vi "File_Write_v2.vi"(0 "Thermocouple Data":dynamicdata(waveform), 1 "Pressure Data":T2, 3 "Flow Rate Data":cluster{dbl, dbl, dbl, dbl, dbl}, 4 "Raman Data Array":cluster{i32[], i32[]}[](array[cluster]), 5 "Loop Iteration Boolean":bool, 8 "File Path Cluster":T3, 9 "Data Cluster":T1={"Current DoE"=[], "SSI 1 Flow Rate"=0.0, "SSI 2 Flow Rate"=0.0, "FLOM 1 Flow Rate"=0.0, "FLOM 2 Flow Rate"=0.0, "Pumps Running?"=FALSE, "Boolean 2"=FALSE, "Boolean 3"=FALSE, "Boolean 4"=FALSE, "At Equilibrium?"=FALSE, "Script Running?"=FALSE, "Current Script Iteration"=0.0, "Total Script Iterations"=0.0, "FLOM Pumps VISA"="COM2", "SSI 1 Pump VISA"="COM76", "SSI 2 Pump VISA"="COM74", "Huber Unistat VISA"="COM1", "SSI 3 Pump VISA"="COM76", "SSI 4 Pump VISA"="COM76", "SSI 4 Flow Rate"=0.0, "SSI 3 Flow Rate"=0.0, "Flow Meter 1"="COM76", "Flow Meter 2"="COM76", "Flow Meter 3"="COM76", "Flow Meter 4"="COM76", "Flow Meter 1 Rate "=0.0, "Flow Meter 2 Rate"=0.0, "Flow Meter 3 Rate"=0.0, "Flow Meter 4 Rate"=0.0, "SSI 1 Flow Setpoint"=0.0, "SSI 2 Flow Setpoint"=0.0, "SSI 3 Flow Setpoint"=0.0, "SSI 4 Flow Setpoint"=0.0, "Temperature Setpoint"=0.0} {"Current DoE" format="%0.3f"}, 12 "Numeric":i32, 13 "Array":i32[](array[numeric])) -> (14 "Data_noRaman path":path, 15 "Data_Reactant 1 path":path caption="selected path", 16 "Data_Reactant 1 path":path, 17 "Data_Reactant 2 path":path caption="selected path", 20 "Data_Reactant 2 path":path, 21 "Data_Reactant 3 path":path, 23 "Data_Product path":path, 24 "Data_noRaman path":path caption="selected path", 25 "Data_Product path":path caption="selected path", 27 "Data_Reactant 3 path":path caption="selected path")   [LabVIEW 2015]
uses:
  --Controls and TypeDefs--/DoE_Control_Cluster.ctl
  <vilib>/Utility/file.llb/Write To Spreadsheet File (string).vi
panel:
  out "appended array":dbl[](array[numeric])
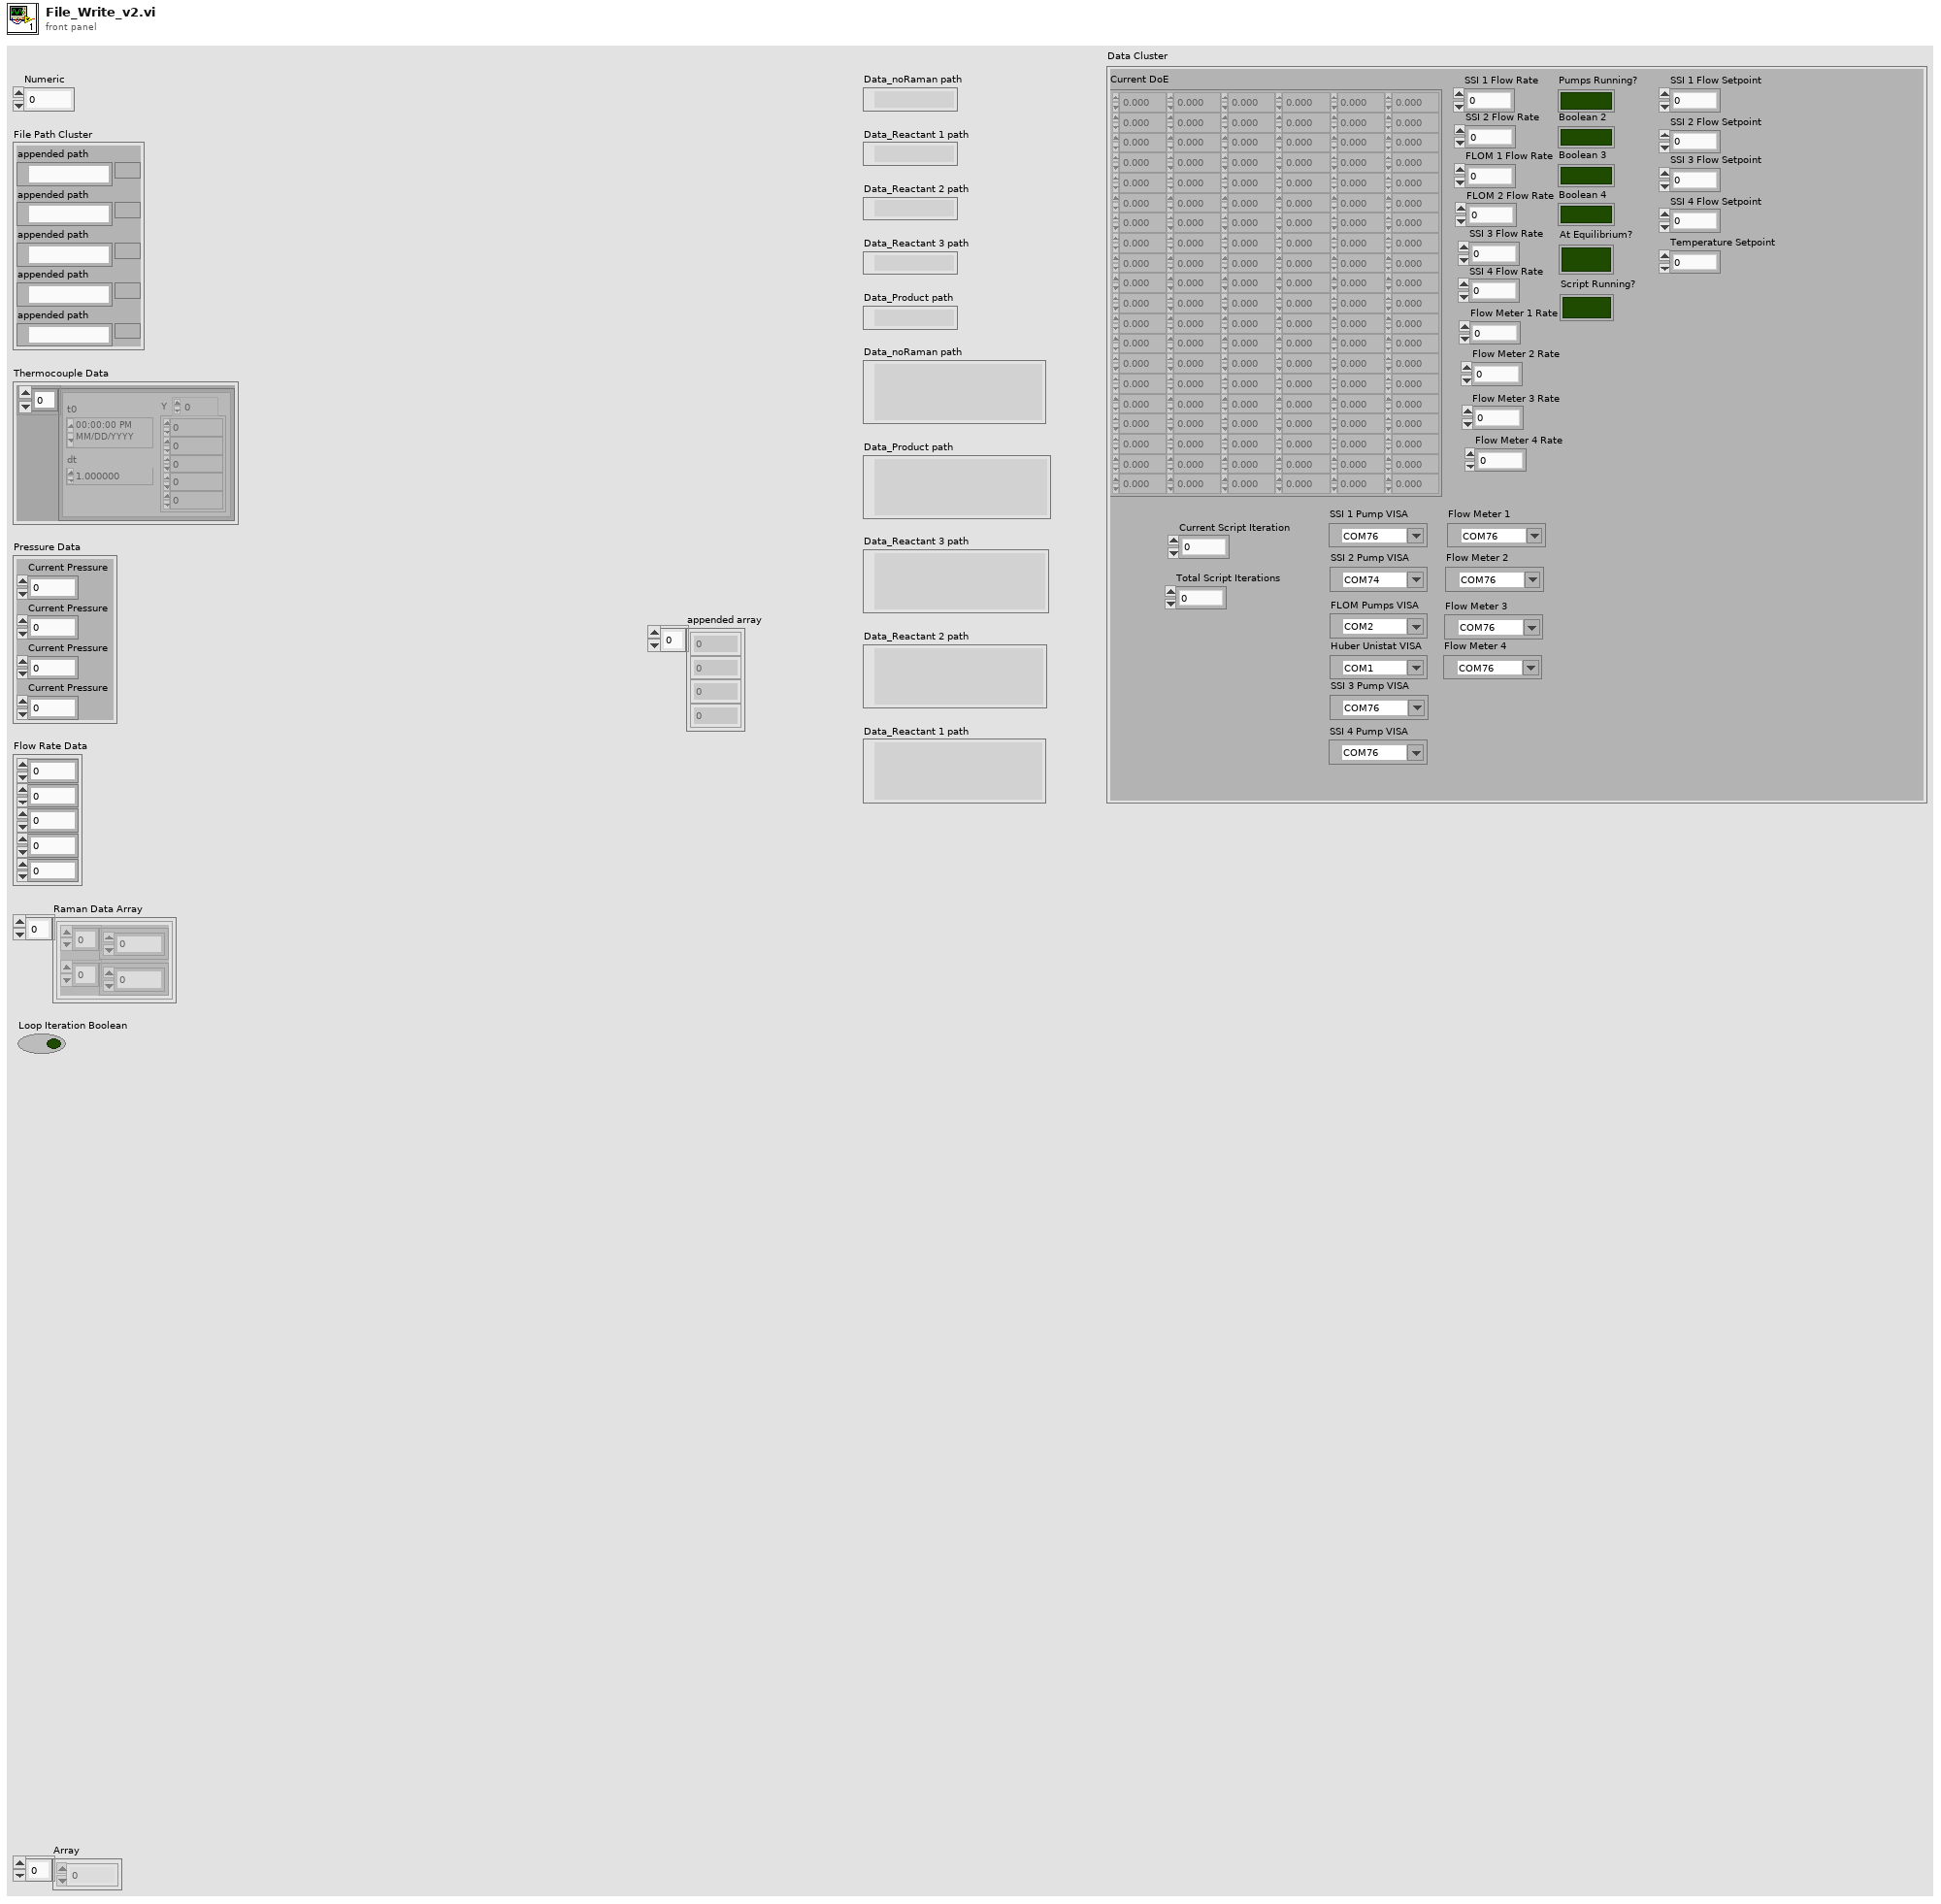
[diagram p1: front panel]
types:
  T1 = typedef "DoE_Control_Cluster.ctl" = cluster{"Current DoE":dbl[][], "SSI 1 Flow Rate":dbl, "SSI 2 Flow Rate":dbl, "FLOM 1 Flow Rate":dbl, "FLOM 2 Flow Rate":dbl, "Pumps Running?":bool, "Boolean 2":bool, "Boolean 3":bool, "Boolean 4":bool, "At Equilibrium?":bool, "Script Running?":bool, "Current Script Iteration":dbl, "Total Script Iterations":dbl, "FLOM Pumps VISA":refnum<visa-resource-name>, "SSI 1 Pump VISA":refnum<visa-resource-name>, "SSI 2 Pump VISA":refnum<visa-resource-name>, "Huber Unistat VISA":refnum<visa-resource-name>, "SSI 3 Pump VISA":refnum<visa-resource-name>, "SSI 4 Pump VISA":refnum<visa-resource-name>, "SSI 4 Flow Rate":dbl, "SSI 3 Flow Rate":dbl, "Flow Meter 1":refnum<visa-resource-name>, "Flow Meter 2":refnum<visa-resource-name>, "Flow Meter 3":refnum<visa-resource-name>, "Flow Meter 4":refnum<visa-resource-name>, "Flow Meter 1 Rate ":dbl, "Flow Meter 2 Rate":dbl, "Flow Meter 3 Rate":dbl, "Flow Meter 4 Rate":dbl, "SSI 1 Flow Setpoint":dbl, "SSI 2 Flow Setpoint":dbl, "SSI 3 Flow Setpoint":dbl, "SSI 4 Flow Setpoint":dbl, "Temperature Setpoint":dbl}
  T2 = cluster{"Current Pressure":dbl, "Current Pressure":dbl, "Current Pressure":dbl, "Current Pressure":dbl}
  T3 = cluster{"appended path":path, "appended path":path, "appended path":path, "appended path":path, "appended path":path}
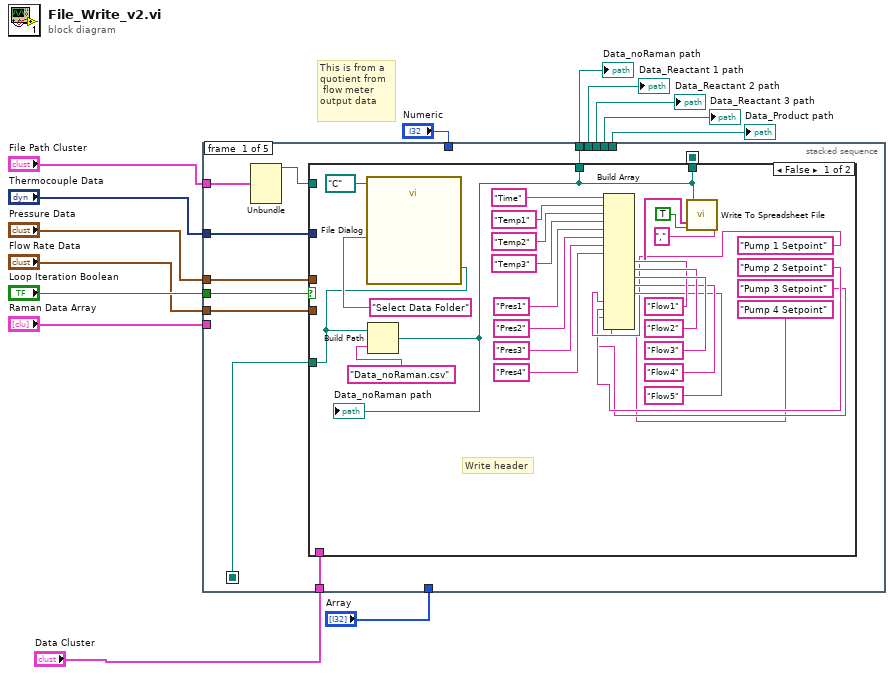
[diagram p0: block diagram]
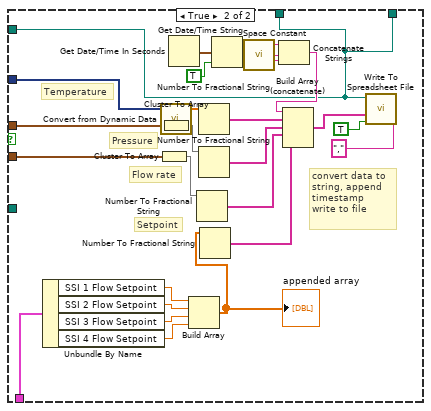
[diagram p2: hidden frame]
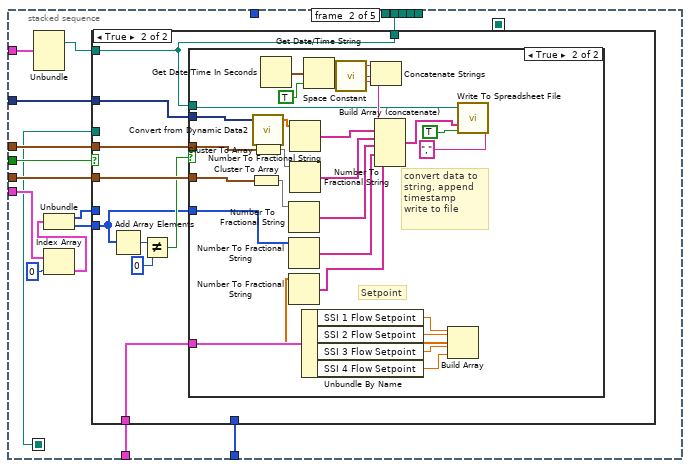
[diagram p3: hidden frame]
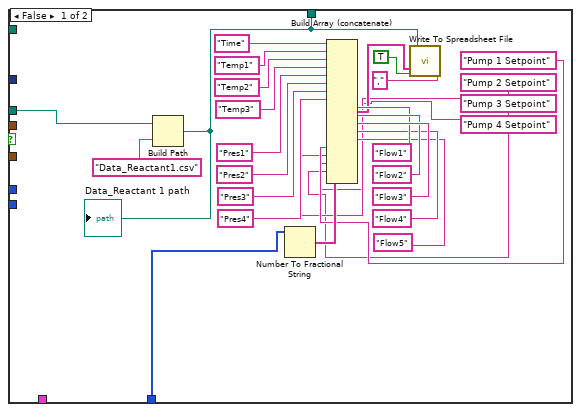
[diagram p4: hidden frame]
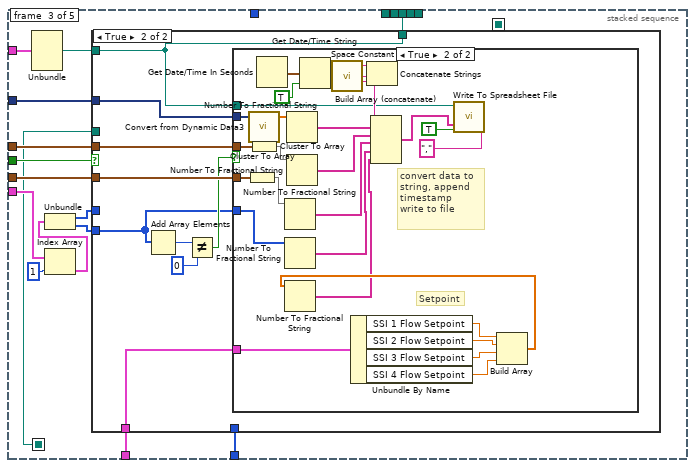
[diagram p6: hidden frame]
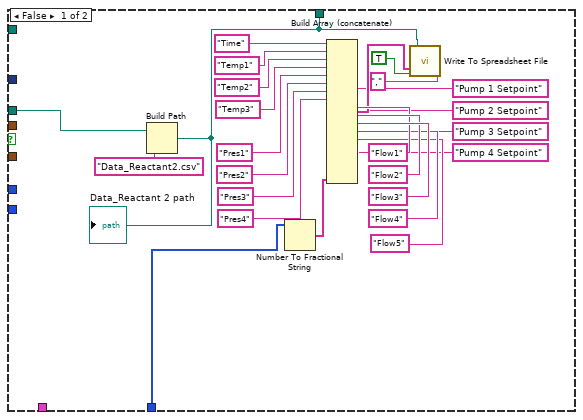
[diagram p7: hidden frame]
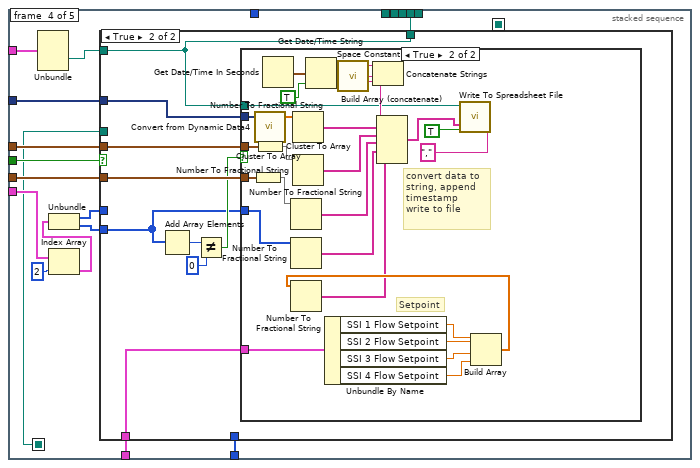
[diagram p9: hidden frame]
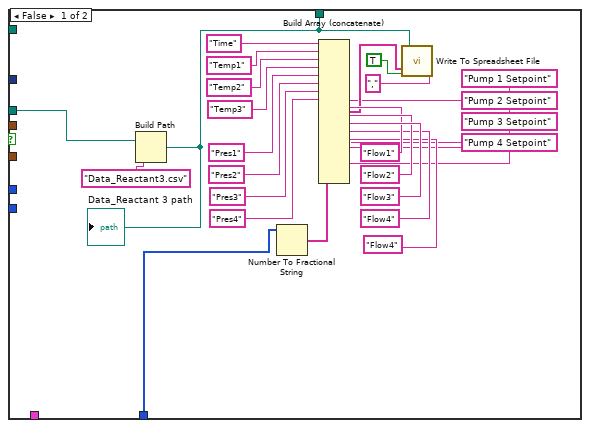
[diagram p10: hidden frame]
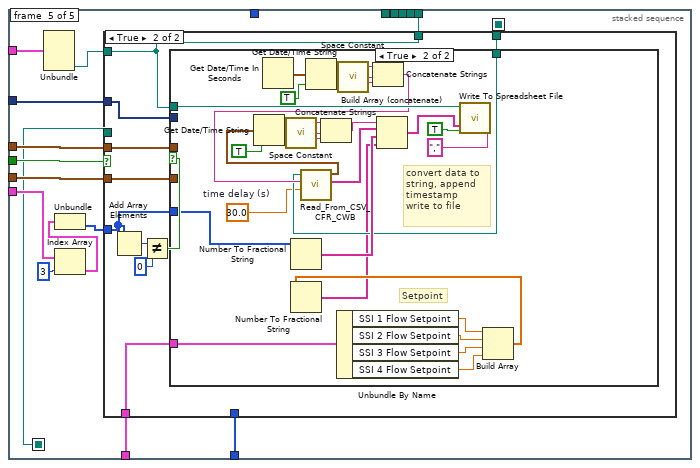
[diagram p12: hidden frame]
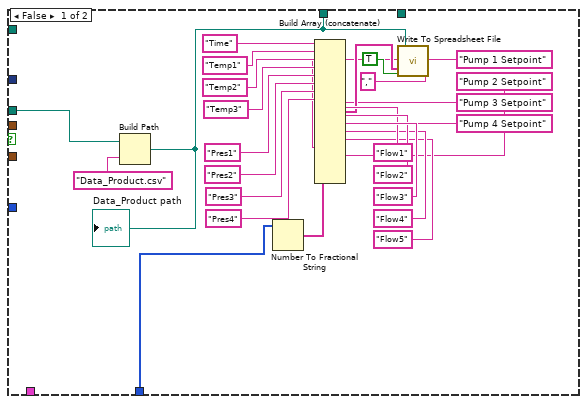
[diagram p13: hidden frame]
diagram:
  # "This is from a \nquotient from\n flow meter\noutput data"
  n1 = stacked-sequence {
    seq-local: [w18 _ _ _ _] -> [_ w78 w155 w232 w310]
    seq-local: [w17 _ _ _ _] -> [_ _ _ _ w308]
    tunnel: "Thermocouple Data" -> [w19 w90 w167 w244 w321]
    tunnel: "Pressure Data" -> [w24 w89 w166 w243 w320]
    tunnel: "Flow Rate Data" -> [w23 w88 w165 w242 w319]
    tunnel: "Loop Iteration Boolean" -> [w22 w87 w164 w241 w318]
    tunnel: [w15 _ _ _ _] -> w12
    tunnel: "File Path Cluster" -> [w21 w80 w157 w234 w312]
    tunnel: "Raman Data Array" -> [_ w84 w161 w238 w316]
    tunnel: [_ w81 _ _ _] -> w11
    tunnel: [_ _ w158 _ _] -> w10
    tunnel: [_ _ _ w235 _] -> w9
    tunnel: [_ _ _ _ w313] -> w8
    tunnel: "Array" -> [_ w77 w154 w231 w309]
    tunnel: "Numeric" -> [_ _ _ _ _]
    tunnel: "Data Cluster" -> [w16 w76 w153 w230 w307]
    frame #0 {
      n2 = Unbundle(w21) -> ("appended path"=w20:path)  [unwired: 4 out]
      n3 = case shown="False" w22 {
        tunnel: w19 -> [_ w63]
        tunnel: w24 -> [_ w62]
        tunnel: w23 -> [_ w59]
        tunnel: w20 -> [_ w57]
        tunnel: [w30 w57] -> w15
        tunnel: [w31 _] -> w18
        tunnel: [w30 w57] -> w17
        tunnel: w16 -> [_ w56]
        frame False {
          # "Write header"
          n4 = call "File Dialog"("start path"=path "C:/", "prompt"="Select Data Folder") -> ("selected path"=w31:path)  [unwired: 10 in, 3 out]
          n5 = Build Path(base path=w31, name or relative path="Data_noRaman.csv" ("default name")) -> (appended path=w30:path)
          "Data_noRaman path" <- w30
          n6 = Build Array("Time" ("delimiter (\\t)"), "Temp1" ("delimiter (\\t)"), "Temp2" ("delimiter (\\t)"), "Temp3" ("delimiter (\\t)"), "Pres1" ("delimiter (\\t)"), "Pres2" ("delimiter (\\t)"), "Pres3" ("delimiter (\\t)"), "Pres4" ("delimiter (\\t)"), "Flow1" ("delimiter (\\t)"), "Flow2" ("delimiter (\\t)"), "Flow3" ("delimiter (\\t)"), "Flow4" ("delimiter (\\t)"), "Flow5" ("delimiter (\\t)"), "Pump 1 Setpoint", "Pump 2 Setpoint", "Pump 3 Setpoint", "Pump 4 Setpoint") -> (w37:string[])
          n7 = call-poly <vilib>:"Write To Spreadsheet File.vi"("delimiter (\\t)"="," ("delimiter (\\t)"), "append to file? (new file:F)"=TRUE ("append to file?"), "1D data"=w37, "file path (dialog if empty)"=w30) -> ()  [unwired: 4 in, 1 out]
        }
        frame True {
          # "Setpoint"
          # "Temperature"
          # "Pressure"
          # "Flow rate"
          # "convert data to \nstring, append\ntimestamp\nwrite to file"
          n8 = Unbundle By Name(w56) -> ("SSI 1 Flow Setpoint"=w55:dbl, "SSI 2 Flow Setpoint"=w54:dbl, "SSI 3 Flow Setpoint"=w53:dbl, "SSI 4 Flow Setpoint"=w52:dbl)
          n9 = Cluster To Array(cluster=w59) -> (array=w60:dbl[])
          n10 = call "Convert from Dynamic Data"("Dynamic Data Type"=w63) -> ("Array"=w72:dbl[])  [unwired: 3 in]
          n11 = Cluster To Array(cluster=w62) -> (array=w73:dbl[])
          n12 = Get Date/Time In Seconds() -> (seconds since 1Jan1904=w66:timestamp)
          n13 = Build Array(w55, w54, w53, w52) -> (w51:dbl[])
          "appended array" <- w51
          n14 = Number To Fractional String(number=w60) -> (F-format string=w58:string[])  [unwired: 3 in]
          n15 = Number To Fractional String(number=w72) -> (F-format string=w74:string[])  [unwired: 3 in]
          n16 = Number To Fractional String(number=w73) -> (F-format string=w61:string[])  [unwired: 3 in]
          n17 = Number To Fractional String(number=w51) -> (F-format string=w50:string[])  [unwired: 3 in]
          n18 = Get Date/Time String(seconds (now)=w66, want seconds? (F)=TRUE) -> (date string=w68:string, time string=w69:string)  [unwired: 1 in]
          n19 = call <vilib>:"Space Constant.vi"() -> ("String"=w70:string)
          n20 = Concatenate Strings(w68, w70, w69) -> (w71:string)
          n21 = Build Array (concatenate)(w71, w74, w61, w58, w50) -> (w75:string[])
          n22 = call-poly <vilib>:"Write To Spreadsheet File.vi"("delimiter (\\t)"="," ("delimiter (\\t)"), "append to file? (new file:F)"=TRUE ("append to file?"), "1D data"=w75, "file path (dialog if empty)"=w57) -> ()  [unwired: 4 in, 1 out]
        }
      }
    }
    frame #1 {
      n23 = Unbundle(w80) -> ("appended path"=w79:path)  [unwired: 4 out]
      n24 = Index Array(array=w84, index=0) -> (element=w83:cluster{i32[], i32[]})
      n25 = Unbundle(w83) -> (w85:i32[], w86:i32[])
      n26 = case shown="True" w87 {
        tunnel: w90 -> [_ w124]
        tunnel: w89 -> [_ w123]
        tunnel: w88 -> [_ w122]
        tunnel: w79 -> [_ w121]
        tunnel: [w115 w121] -> w81
        tunnel: w86 -> [_ w117]
        tunnel: w85 -> [_ _]
        tunnel: w78 -> [w114 _]
        tunnel: w77 -> [w97 _]
        tunnel: w76 -> [_ w116]
        frame False {
          n27 = Build Path(base path=w114, name or relative path="Data_Reactant1.csv" ("default name")) -> (appended path=w115:path)
          "Data_Reactant 1 path" <- w115
          n28 = Number To Fractional String(number=w97) -> (F-format string=w95:string[])  [unwired: 3 in]
          n29 = Build Array (concatenate)("Time" ("delimiter (\\t)"), "Temp1" ("delimiter (\\t)"), "Temp2" ("delimiter (\\t)"), "Temp3" ("delimiter (\\t)"), "Pres1" ("delimiter (\\t)"), "Pres2" ("delimiter (\\t)"), "Pres3" ("delimiter (\\t)"), "Pres4" ("delimiter (\\t)"), "Flow1" ("delimiter (\\t)"), "Flow2" ("delimiter (\\t)"), "Flow3" ("delimiter (\\t)"), "Flow4" ("delimiter (\\t)"), "Flow5" ("delimiter (\\t)"), "Pump 1 Setpoint", "Pump 2 Setpoint", "Pump 3 Setpoint", "Pump 4 Setpoint", w95) -> (w101:string[])
          n30 = call-poly <vilib>:"Write To Spreadsheet File.vi"("delimiter (\\t)"="," ("delimiter (\\t)"), "append to file? (new file:F)"=TRUE ("append to file?"), "1D data"=w101, "file path (dialog if empty)"=w115) -> ()  [unwired: 4 in, 1 out]
        }
        frame True {
          n31 = Add Array Elements(numeric array=w117) -> (sum=w120:i32)
          n32 = Not Equal?(x=w120, y=0) -> (x != y?=w118:bool)
          n33 = case shown="True" w118 {
            tunnel: w124 -> [_ w140]
            tunnel: w123 -> [_ w139]
            tunnel: w122 -> [_ w136]
            tunnel: w121 -> [_ w134]
            tunnel: w117 -> [_ w133]
            tunnel: w116 -> [_ w128]
            frame False {
            }
            frame True {
              # "Setpoint"
              # "convert data to \nstring, append\ntimestamp\nwrite to file"
              n34 = Cluster To Array(cluster=w136) -> (array=w137:dbl[])
              n35 = call "Convert from Dynamic Data2"("Dynamic Data Type"=w140) -> ("Array"=w149:dbl[])  [unwired: 3 in]
              n36 = Cluster To Array(cluster=w139) -> (array=w150:dbl[])
              n37 = Get Date/Time In Seconds() -> (seconds since 1Jan1904=w143:timestamp)
              n38 = Number To Fractional String(number=w137) -> (F-format string=w135:string[])  [unwired: 3 in]
              n39 = Number To Fractional String(number=w133) -> (F-format string=w132:string[])  [unwired: 3 in]
              n40 = Number To Fractional String(number=w149) -> (F-format string=w151:string[])  [unwired: 3 in]
              n41 = Number To Fractional String(number=w150) -> (F-format string=w138:string[])  [unwired: 3 in]
              n42 = Unbundle By Name(w128) -> ("SSI 1 Flow Setpoint"=w131:dbl, "SSI 2 Flow Setpoint"=w127:dbl, "SSI 3 Flow Setpoint"=w130:dbl, "SSI 4 Flow Setpoint"=w129:dbl)
              n43 = Get Date/Time String(seconds (now)=w143, want seconds? (F)=TRUE) -> (date string=w145:string, time string=w146:string)  [unwired: 1 in]
              n44 = call <vilib>:"Space Constant.vi"() -> ("String"=w147:string)
              n45 = Concatenate Strings(w145, w147, w146) -> (w148:string)
              n46 = Build Array(w131, w127, w130, w129) -> (w126:dbl[])
              n47 = Number To Fractional String(number=w126) -> (F-format string=w125:string[])  [unwired: 3 in]
              n48 = Build Array (concatenate)(w148, w151, w138, w135, w132, w125) -> (w152:string[])
              n49 = call-poly <vilib>:"Write To Spreadsheet File.vi"("delimiter (\\t)"="," ("delimiter (\\t)"), "append to file? (new file:F)"=TRUE ("append to file?"), "1D data"=w152, "file path (dialog if empty)"=w134) -> ()  [unwired: 4 in, 1 out]
            }
          }
        }
      }
    }
    frame #2 {
      n50 = Unbundle(w157) -> ("appended path"=w156:path)  [unwired: 4 out]
      n51 = Index Array(array=w161, index=1) -> (element=w160:cluster{i32[], i32[]})
      n52 = Unbundle(w160) -> (w162:i32[], w163:i32[])
      n53 = case shown="True" w164 {
        tunnel: w167 -> [_ w201]
        tunnel: w166 -> [_ w200]
        tunnel: w165 -> [_ w199]
        tunnel: w156 -> [_ w198]
        tunnel: [w192 w198] -> w158
        tunnel: w163 -> [_ w194]
        tunnel: w162 -> [_ _]
        tunnel: w155 -> [w191 _]
        tunnel: w154 -> [w174 _]
        tunnel: w153 -> [_ w193]
        frame False {
          n54 = Build Path(base path=w191, name or relative path="Data_Reactant2.csv" ("default name")) -> (appended path=w192:path)
          "Data_Reactant 2 path" <- w192
          n55 = Number To Fractional String(number=w174) -> (F-format string=w172:string[])  [unwired: 3 in]
          n56 = Build Array (concatenate)("Time" ("delimiter (\\t)"), "Temp1" ("delimiter (\\t)"), "Temp2" ("delimiter (\\t)"), "Temp3" ("delimiter (\\t)"), "Pres1" ("delimiter (\\t)"), "Pres2" ("delimiter (\\t)"), "Pres3" ("delimiter (\\t)"), "Pres4" ("delimiter (\\t)"), "Flow1" ("delimiter (\\t)"), "Flow2" ("delimiter (\\t)"), "Flow3" ("delimiter (\\t)"), "Flow4" ("delimiter (\\t)"), "Flow5" ("delimiter (\\t)"), "Pump 1 Setpoint", "Pump 2 Setpoint", "Pump 3 Setpoint", "Pump 4 Setpoint", w172) -> (w178:string[])
          n57 = call-poly <vilib>:"Write To Spreadsheet File.vi"("delimiter (\\t)"="," ("delimiter (\\t)"), "append to file? (new file:F)"=TRUE ("append to file?"), "1D data"=w178, "file path (dialog if empty)"=w192) -> ()  [unwired: 4 in, 1 out]
        }
        frame True {
          n58 = Add Array Elements(numeric array=w194) -> (sum=w197:i32)
          n59 = Not Equal?(x=w197, y=0) -> (x != y?=w195:bool)
          n60 = case shown="True" w195 {
            tunnel: w201 -> [_ w217]
            tunnel: w200 -> [_ w216]
            tunnel: w199 -> [_ w213]
            tunnel: w198 -> [_ w211]
            tunnel: w194 -> [_ w210]
            tunnel: w193 -> [_ w205]
            frame False {
            }
            frame True {
              # "Setpoint"
              # "convert data to \nstring, append\ntimestamp\nwrite to file"
              n61 = Cluster To Array(cluster=w213) -> (array=w214:dbl[])
              n62 = call "Convert from Dynamic Data3"("Dynamic Data Type"=w217) -> ("Array"=w226:dbl[])  [unwired: 3 in]
              n63 = Cluster To Array(cluster=w216) -> (array=w227:dbl[])
              n64 = Get Date/Time In Seconds() -> (seconds since 1Jan1904=w220:timestamp)
              n65 = Number To Fractional String(number=w214) -> (F-format string=w212:string[])  [unwired: 3 in]
              n66 = Number To Fractional String(number=w210) -> (F-format string=w209:string[])  [unwired: 3 in]
              n67 = Number To Fractional String(number=w226) -> (F-format string=w228:string[])  [unwired: 3 in]
              n68 = Number To Fractional String(number=w227) -> (F-format string=w215:string[])  [unwired: 3 in]
              n69 = Get Date/Time String(seconds (now)=w220, want seconds? (F)=TRUE) -> (date string=w222:string, time string=w223:string)  [unwired: 1 in]
              n70 = call <vilib>:"Space Constant.vi"() -> ("String"=w224:string)
              n71 = Unbundle By Name(w205) -> ("SSI 1 Flow Setpoint"=w208:dbl, "SSI 2 Flow Setpoint"=w204:dbl, "SSI 3 Flow Setpoint"=w207:dbl, "SSI 4 Flow Setpoint"=w206:dbl)
              n72 = Concatenate Strings(w222, w224, w223) -> (w225:string)
              n73 = Build Array(w208, w204, w207, w206) -> (w203:dbl[])
              n74 = Number To Fractional String(number=w203) -> (F-format string=w202:string[])  [unwired: 3 in]
              n75 = Build Array (concatenate)(w225, w228, w215, w212, w209, w202) -> (w229:string[])
              n76 = call-poly <vilib>:"Write To Spreadsheet File.vi"("delimiter (\\t)"="," ("delimiter (\\t)"), "append to file? (new file:F)"=TRUE ("append to file?"), "1D data"=w229, "file path (dialog if empty)"=w211) -> ()  [unwired: 4 in, 1 out]
            }
          }
        }
      }
    }
    frame #3 {
      n77 = Unbundle(w234) -> ("appended path"=w233:path)  [unwired: 4 out]
      n78 = Index Array(array=w238, index=2) -> (element=w237:cluster{i32[], i32[]})
      n79 = Unbundle(w237) -> (w239:i32[], w240:i32[])
      n80 = case shown="True" w241 {
        tunnel: w244 -> [_ w278]
        tunnel: w243 -> [_ w277]
        tunnel: w242 -> [_ w276]
        tunnel: w233 -> [_ w275]
        tunnel: [w269 w275] -> w235
        tunnel: w240 -> [_ w271]
        tunnel: w239 -> [_ _]
        tunnel: w232 -> [w268 _]
        tunnel: w231 -> [w251 _]
        tunnel: w230 -> [_ w270]
        frame False {
          n81 = Build Path(base path=w268, name or relative path="Data_Reactant3.csv" ("default name")) -> (appended path=w269:path)
          "Data_Reactant 3 path" <- w269
          n82 = Number To Fractional String(number=w251) -> (F-format string=w249:string[])  [unwired: 3 in]
          n83 = Build Array (concatenate)("Time" ("delimiter (\\t)"), "Temp1" ("delimiter (\\t)"), "Temp2" ("delimiter (\\t)"), "Temp3" ("delimiter (\\t)"), "Pres1" ("delimiter (\\t)"), "Pres2" ("delimiter (\\t)"), "Pres3" ("delimiter (\\t)"), "Pres4" ("delimiter (\\t)"), "Flow1" ("delimiter (\\t)"), "Flow2" ("delimiter (\\t)"), "Flow3" ("delimiter (\\t)"), "Flow4" ("delimiter (\\t)"), "Flow4" ("delimiter (\\t)"), "Pump 1 Setpoint", "Pump 2 Setpoint", "Pump 3 Setpoint", "Pump 4 Setpoint", w249) -> (w255:string[])
          n84 = call-poly <vilib>:"Write To Spreadsheet File.vi"("delimiter (\\t)"="," ("delimiter (\\t)"), "append to file? (new file:F)"=TRUE ("append to file?"), "1D data"=w255, "file path (dialog if empty)"=w269) -> ()  [unwired: 4 in, 1 out]
        }
        frame True {
          n85 = Add Array Elements(numeric array=w271) -> (sum=w274:i32)
          n86 = Not Equal?(x=w274, y=0) -> (x != y?=w272:bool)
          n87 = case shown="True" w272 {
            tunnel: w278 -> [_ w294]
            tunnel: w277 -> [_ w293]
            tunnel: w276 -> [_ w290]
            tunnel: w275 -> [_ w288]
            tunnel: w271 -> [_ w287]
            tunnel: w270 -> [_ w282]
            frame False {
            }
            frame True {
              # "Setpoint"
              # "convert data to \nstring, append\ntimestamp\nwrite to file"
              n88 = Cluster To Array(cluster=w290) -> (array=w291:dbl[])
              n89 = call "Convert from Dynamic Data4"("Dynamic Data Type"=w294) -> ("Array"=w303:dbl[])  [unwired: 3 in]
              n90 = Cluster To Array(cluster=w293) -> (array=w304:dbl[])
              n91 = Get Date/Time In Seconds() -> (seconds since 1Jan1904=w297:timestamp)
              n92 = Number To Fractional String(number=w291) -> (F-format string=w289:string[])  [unwired: 3 in]
              n93 = Number To Fractional String(number=w287) -> (F-format string=w286:string[])  [unwired: 3 in]
              n94 = Number To Fractional String(number=w303) -> (F-format string=w305:string[])  [unwired: 3 in]
              n95 = Number To Fractional String(number=w304) -> (F-format string=w292:string[])  [unwired: 3 in]
              n96 = Get Date/Time String(seconds (now)=w297, want seconds? (F)=TRUE) -> (date string=w299:string, time string=w300:string)  [unwired: 1 in]
              n97 = Unbundle By Name(w282) -> ("SSI 1 Flow Setpoint"=w285:dbl, "SSI 2 Flow Setpoint"=w279:dbl, "SSI 3 Flow Setpoint"=w284:dbl, "SSI 4 Flow Setpoint"=w283:dbl)
              n98 = call <vilib>:"Space Constant.vi"() -> ("String"=w301:string)
              n99 = Concatenate Strings(w299, w301, w300) -> (w302:string)
              n100 = Build Array(w285, w279, w284, w283) -> (w281:dbl[])
              n101 = Number To Fractional String(number=w281) -> (F-format string=w280:string[])  [unwired: 3 in]
              n102 = Build Array (concatenate)(w302, w305, w292, w289, w286, w280) -> (w306:string[])
              n103 = call-poly <vilib>:"Write To Spreadsheet File.vi"("delimiter (\\t)"="," ("delimiter (\\t)"), "append to file? (new file:F)"=TRUE ("append to file?"), "1D data"=w306, "file path (dialog if empty)"=w288) -> ()  [unwired: 4 in, 1 out]
            }
          }
        }
      }
    }
    frame #4 {
      n104 = Unbundle(w312) -> ("appended path"=w311:path)  [unwired: 4 out]
      n105 = Index Array(array=w316, index=3) -> (element=w315:cluster{i32[], i32[]})
      n106 = Unbundle(w315) -> (w317:i32[])  [unwired: 1 out]
      n107 = case shown="True" w318 {
        tunnel: w321 -> [_ w356]
        tunnel: w320 -> [_ w355]
        tunnel: w319 -> [_ w354]
        tunnel: w311 -> [_ w348]
        tunnel: [w346 w348] -> w313
        tunnel: w317 -> [_ w350]
        tunnel: w310 -> [w345 _]
        tunnel: w309 -> [w328 _]
        tunnel: w308 -> [_ w349]
        tunnel: w307 -> [_ w347]
        frame False {
          n108 = Build Path(base path=w345, name or relative path="Data_Product.csv" ("default name")) -> (appended path=w346:path)
          "Data_Product path" <- w346
          n109 = Number To Fractional String(number=w328) -> (F-format string=w326:string[])  [unwired: 3 in]
          n110 = Build Array (concatenate)("Time" ("delimiter (\\t)"), "Temp1" ("delimiter (\\t)"), "Temp2" ("delimiter (\\t)"), "Temp3" ("delimiter (\\t)"), "Pres1" ("delimiter (\\t)"), "Pres2" ("delimiter (\\t)"), "Pres3" ("delimiter (\\t)"), "Pres4" ("delimiter (\\t)"), "Flow1" ("delimiter (\\t)"), "Flow2" ("delimiter (\\t)"), "Flow3" ("delimiter (\\t)"), "Flow4" ("delimiter (\\t)"), "Flow5" ("delimiter (\\t)"), "Pump 1 Setpoint", "Pump 2 Setpoint", "Pump 3 Setpoint", "Pump 4 Setpoint", w326) -> (w332:string[])
          n111 = call-poly <vilib>:"Write To Spreadsheet File.vi"("delimiter (\\t)"="," ("delimiter (\\t)"), "append to file? (new file:F)"=TRUE ("append to file?"), "1D data"=w332, "file path (dialog if empty)"=w346) -> ()  [unwired: 4 in, 1 out]
        }
        frame True {
          n112 = Add Array Elements(numeric array=w350) -> (sum=w353:i32)
          n113 = Not Equal?(x=w353, y=0) -> (x != y?=w351:bool)
          n114 = case shown="True" w351 {
            tunnel: w356 -> [_ _]
            tunnel: w355 -> [_ _]
            tunnel: w354 -> [_ _]
            tunnel: w348 -> [_ w376]
            tunnel: w350 -> [_ w375]
            tunnel: w349 -> [_ w366]
            tunnel: w347 -> [_ w360]
            frame False {
            }
            frame True {
              w365 = 30.0  # time delay (s)
              # "Setpoint"
              # "convert data to \nstring, append\ntimestamp\nwrite to file"
              n115 = Get Date/Time In Seconds() -> (seconds since 1Jan1904=w379:timestamp)
              n116 = call <vilib>:"Space Constant.vi"() -> ("String"=w373:string)
              n117 = Number To Fractional String(number=w375) -> (F-format string=w367:string[])  [unwired: 3 in]
              n118 = Get Date/Time String(seconds (now)=w379, want seconds? (F)=TRUE) -> (date string=w381:string, time string=w382:string)  [unwired: 1 in]
              n119 = Unbundle By Name(w360) -> ("SSI 1 Flow Setpoint"=w363:dbl, "SSI 2 Flow Setpoint"=w359:dbl, "SSI 3 Flow Setpoint"=w362:dbl, "SSI 4 Flow Setpoint"=w361:dbl)
              n120 = call <vilib>:"Space Constant.vi"() -> ("String"=w383:string)
              n121 = Concatenate Strings(w381, w383, w382) -> (w374:string)
              n122 = call "Read_From_CSV_CFR_CWB.vi"("time delay (s)"=w365, "input string"=w374, "Spreadsheet path (.csv)"=w366) -> ("output data"=w368:string[], "time stamp"=w370:timestamp)  [unwired: 6 in]
              n123 = Get Date/Time String(seconds (now)=w370, want seconds? (F)=TRUE) -> (date string=w364:string, time string=w372:string)  [unwired: 1 in]
              n124 = Concatenate Strings(w364, w373, w372) -> (w369:string)
              n125 = Build Array(w363, w359, w362, w361) -> (w358:dbl[])
              n126 = Number To Fractional String(number=w358) -> (F-format string=w357:string[])  [unwired: 3 in]
              n127 = Build Array (concatenate)(w369, w368, w367, w357) -> (w384:string[])
              n128 = call-poly <vilib>:"Write To Spreadsheet File.vi"("delimiter (\\t)"="," ("delimiter (\\t)"), "append to file? (new file:F)"=TRUE ("append to file?"), "1D data"=w384, "file path (dialog if empty)"=w376) -> ()  [unwired: 4 in, 1 out]
            }
          }
        }
      }
    }
  }
  "Data_noRaman path" <- w12
  "Data_Reactant 1 path" <- w11
  "Data_Reactant 2 path" <- w10
  "Data_Reactant 3 path" <- w9
  "Data_Product path" <- w8
